vi "Laurel Modbus Reset Total.vi"(8 "Error In":errorcluster, 11 "Modbus Master in":refnum<class "Modbus Master.lvclass">) -> (0 "Error Out":errorcluster, 3 "Modbus Master out":refnum<class "Modbus Master.lvclass">)   [LabVIEW 2020]
uses:
  <vilib>/NI/Modbus Library/API/Master/Modbus Master.lvclass
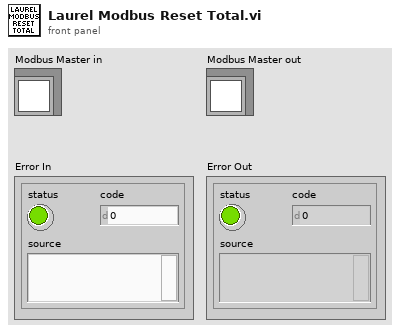
[diagram p1: front panel]
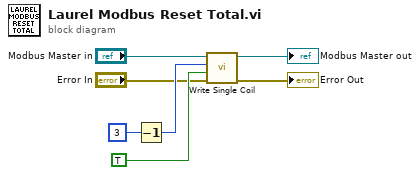
[diagram p0: block diagram]
diagram:
  n1 = Decrement(x=u16 3 ("starting address 2")) -> (x-1=w6:u16)
  n2 = call-dynamic "Write Single Coil.vi"("error in"="Error In", "coil to write"=TRUE, "address"=w6, "Modbus master in"="Modbus Master in") -> ("error out"=→"Error Out":errorcluster, "Modbus master out"=→"Modbus Master out":refnum<class "Modbus Master.lvclass">)  [unwired: 6 in]
